vi "Beam_Check_Titles.vi"() -> (0 "Titles":string[](array[string])=["Number:Of:Traverses", "Laser:Beam:Type", "Trav:Name:1", "X:Traverse:1", "Y:Traverse:1", "Z:Traverse:1", "Trav:Name:2", "X:Traverse:2", "Y:Traverse:2", "Z:Traverse:2"])   [LabVIEW 2020]
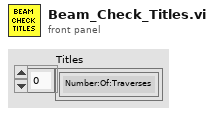
[diagram p1: front panel]
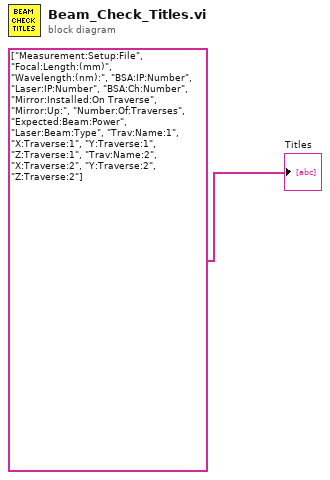
[diagram p0: block diagram]
diagram:
  "Titles" <- string[] ["Measurement:Setup:File", "Focal:Length:(mm)", "Wavelength:(nm):", "BSA:IP:Number", "Laser:IP:Number", "BSA:Ch:Number", "Mirror:Installed:On Traverse", "Mirror:Up:", "Number:Of:Traverses", "Expected:Beam:Power", "Laser:Beam:Type", "Trav:Name:1", "X:Traverse:1", "Y:Traverse:1", "Z:Traverse:1", "Trav:Name:2", "X:Traverse:2", "Y:Traverse:2", "Z:Traverse:2"] ("appended array")
